vi "roboRIO v1.0 Open Accelerometer.vi"(7 "Allow multiple opens?":bool, 8 "error in (no error)":errorcluster, 10 "Channel Names":string[](array[string]), 11 "Resource name":T3 caption="RIO Device") -> (0 "error out":errorcluster, 1 "LSB Weight":dbl, 2 "Accelerometer Channel List":T4, 3 "myRIO Ref Out":T1)   [LabVIEW 2021]
uses:
  <vilib>/myRIO/Common/Instrument Driver Framework/myRIO v1.0/Accelerometer/typedefs/Accelerometer Channels List.ctl
  <vilib>/myRIO/Common/Instrument Driver Framework/myRIO v1.0/Accelerometer/typedefs/Accelerometer Channels Enum.ctl
  <vilib>/userDefined/High Color/nirio_resource_hc.ctl
  <vilib>/myRIO/Common/Instrument Driver Framework/Utilities/typedefs/myRIO v1.0 Reference.ctl
  <vilib>/myRIO/Common/Instrument Driver Framework/Utilities/typedefs/Generic FPGA Reference.ctl
  <vilib>/myRIO/Common/Instrument Driver Framework/roboRIO v1.0/Accelerometer/typedefs/roboRIO Accelerometer Channels Enum.ctl
  <vilib>/myRIO/Common/Instrument Driver Framework/roboRIO v1.0/Resource Manager/vis/roboRIO v1.0 Reserve Channel List.vi
  <vilib>/myRIO/Common/Instrument Driver Framework/roboRIO v1.0/Accelerometer/vis/roboRIO v1.0 Build MUX Configuration Accelerometer.vi
  <vilib>/myRIO/Common/Instrument Driver Framework/roboRIO v1.0/Resource Manager/vis/roboRIO v1.0 Reserve Channel.vi
  <vilib>/myRIO/Common/Instrument Driver Framework/roboRIO v1.0/Resource Manager/vis/roboRIO v1.0 Unreserve Channel.vi
  <vilib>/myRIO/Common/Instrument Driver Framework/roboRIO v1.0/Resource Manager/vis/roboRIO v1.0 Build Mutex Name.vi
  <vilib>/Utility/VariantDataType/GetNumericInfo.vi
  <vilib>/Utility/error.llb/Error Cluster From Error Code.vi
  <vilib>/myRIO/Common/Instrument Driver Framework/Utilities/vis/IO Manager.vi
  <vilib>/myRIO/Common/Instrument Driver Framework/Utilities/vis/Configuration Manager.vi
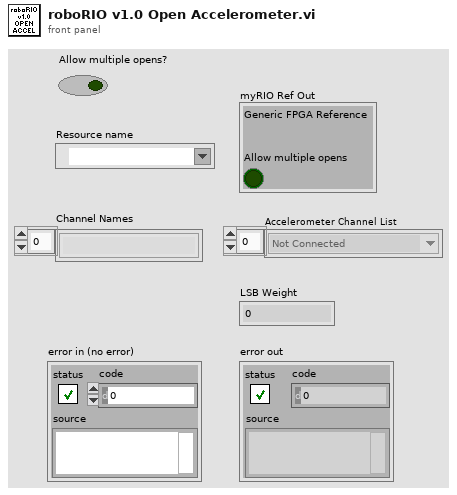
[diagram p1: front panel]
types:
  T1 = typedef "myRIO v1.0 Reference.ctl" = cluster{"Generic FPGA Reference":T2, "Allow multiple opens":bool}
  T2 = typedef "Generic FPGA Reference.ctl" = refnum<k20>
  T3 = typedef "nirio_resource_hc.ctl" = tag
  T4 = typedef "Accelerometer Channels List.ctl" = T5[]
  T5 = typedef "Accelerometer Channels Enum.ctl" = enum16{"Not Connected", "X-Axis", "Y-Axis", "Z-Axis"}
  T6 = typedef "roboRIO Accelerometer Channels Enum.ctl" = enum16{"Not Connected", "X-Axis", "Y-Axis", "Z-Axis"}
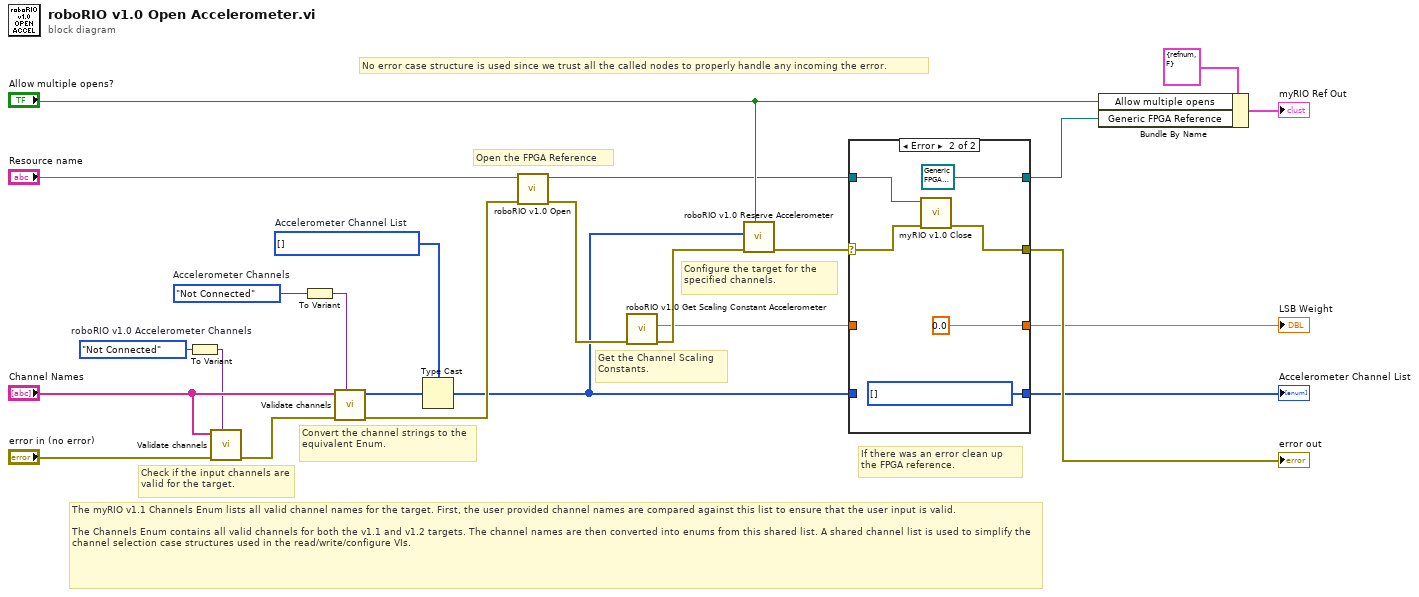
[diagram p0: block diagram]
diagram:
  w8 = roboRIO_Accelerometer_Channels_Enum."Not Connected"  # roboRIO v1.0 Accelerometer Channels
  w7 = Accelerometer_Channels_Enum."Not Connected"  # Accelerometer Channels
  w18 = T4 [] items=["Not Connected", "X-Axis", "Y-Axis", "Z-Axis"]  # Accelerometer Channel List
  # "Get the Channel Scaling Constants."
  # "The myRIO v1.1 Channels Enum lists all valid channel names for the target. First, the user provided channel names are compared against this list to ensure that the user input is valid.\n\nThe Channels Enum contains all valid channels for both the v1.1 and v1.2 targets. The channel names are then converted into enums from this shared list. A shared channel list is used to simplify the channel selection case structures used in the read/write/configure VIs."
  # "If there was an error clean up the FPGA reference."
  # "Configure the target for the specified channels."
  # "Open the FPGA Reference"
  # "No error case structure is used since we trust all the called nodes to properly handle any incoming the error."
  # "Convert the channel strings to the equivalent Enum."
  # "Check if the input channels are valid for the target."
  n1 = To Variant(anything=w8) -> (Variant=w9:variant)
  n2 = call <vilib>:"Validate channels.vi"("Channels Enum Variant"=w9, "error in (no error)"="error in (no error)", "Channel Names"="Channel Names") -> ("error out"=w23:errorcluster)  [unwired: 7 in, 1 out]
  n3 = To Variant(anything=w7) -> (Variant=w10:variant)
  n4 = call <vilib>:"Validate channels.vi"("Channels Enum Variant"=w10, "error in (no error)"=w23, "Channel Names"="Channel Names") -> ("error out"=w19:errorcluster, "Index Array"=w17:u16[])  [unwired: 7 in]
  n5 = Type Cast(type=w18, x=w17) -> (*(type *) &x=w5:T4)
  n6 = call <vilib>:"roboRIO v1.0 Open.vi"("error in (no error)"=w19, "Resource name"="Resource name") -> ("error out"=w6:errorcluster, "myRIO FPGA Ref Out"=w4:T2)  [unwired: 8 in]
  n7 = call <vilib>:"roboRIO v1.0 Get Scaling Constant Accelerometer.vi"("error in (no error)"=w6) -> ("error out"=w3:errorcluster, "LSB Weight (g-force/bit)"=w2:dbl)  [unwired: 9 in]
  n8 = call <vilib>:"roboRIO v1.0 Reserve Accelerometer.vi"("Allow multiple opens?"="Allow multiple opens?", "error in (no error)"=w3, "AI Channel List"=w5) -> ("error out"=w16:errorcluster)  [unwired: 8 in]
  n9 = case shown="Error" w16 {
    selector: w16 -> [w27 w34]
    tunnel: w4 -> [w28 w32]
    tunnel: [w28 T2 refnum ("myRIO FPGA Ref Out")] -> w12
    tunnel: [w27 w33] -> w21
    tunnel: [w26 w30] -> w15
    tunnel: w5 -> [w26 _]
    tunnel: w2 -> [w25 _]
    tunnel: [w25 0.0 ("LSB Weight")] -> w1
    frame No Error {
    }
    frame Error {
      w30 = T4 [] items=["Not Connected", "X-Axis", "Y-Axis", "Z-Axis"]
      n10 = call <vilib>:"myRIO v1.0 Close.vi"("error in (no error)"=w34, "myRIO FPGA Ref In"=w32) -> ("error out"=w33:errorcluster)  [unwired: 9 in]
    }
  }
  "Accelerometer Channel List" <- w15
  "error out" <- w21
  "LSB Weight" <- w1
  n11 = Bundle By Name(cluster=T1 {"Generic FPGA Reference"=refnum, "Allow multiple opens"=FALSE} ("myRIO Hardware Reference"), "Allow multiple opens"="Allow multiple opens?", "Generic FPGA Reference"=w12) -> (→"myRIO Ref Out":T1)
